vi "GUI PJVS setup.vi"(10 "SS measurement":T1={"Signal frequencies (Hz)"=[1000.0], "Signal amplitudes (V)"=[0.707], "Sampling frequencies (Hz)"=[10000000.0], "Record lengths (multiples of periods)"=[10000.0], "Calculate results"=FALSE, "Algorithm"="TWM-WFFT", "TWM data directories"=[], "TWM data directories relative"=[], "Settle down after AC source change (s)"=1.0, "PJVS frequencies (Hz)"=[1000.0], "PJVS reference voltages array of vector cluster"=[{"PJVS reference voltages vector"=[]}], "Requested PJVS steps"=[20], "Measure CE"=FALSE, "Measure CE before"=FALSE, "Measure CE after"=FALSE, "Single point CE measurement"=FALSE, "original CE template path"=path "", "new CE template path before SS"=path "", "new CE template path before SS relative"=path "", "new CE template path after SS"=path "", "new CE template path after SS relative"=path "", "original CE fit path"=path "", "new CE fit path before SS"=path "", "new CE fit path before SS relative"=path "", "new CE fit path after SS"=path "", "new CE fit path after SS relative"=path "", "Measure digitizer gain"=FALSE, "Measure digitizer gain before"=FALSE, "Measure digitizer gain after"=FALSE, "Digitizer gain"=0.0, "Data folder"=path "", "FR fit path"=path "", "new FR fit path relative"=path "", "Rs"=0, "Re"=0, "SS measurement info files"=[]} {"PJVS reference voltages array of vector cluster"."PJVS reference voltages vector" format="%#_3p"; "PJVS frequencies (Hz)" format="%#_3p"; "Record lengths (multiples of periods)" format="%#_3p"; "Sampling frequencies (Hz)" format="%#_3p"; "Signal amplitudes (V)" format="%#_3p"; "Signal frequencies (Hz)" format="%#_3p"}, 11 "PJVS":T2={"PJVS type"=enum."AC-supraVOLTcontrol", "Status Refnum"=refnum, "AC-supraVOLTcontrol"={"IP address:port (0.0.0.0:0000)"="0.0.0.0:0000", "Timeouts"={"TCP Read & Write (ms)"=7000, "Sensors readout"=5000, "PJVS setup"=10000, "Nullmeter readout"=5000, "Multiplexer setup"=3000, "57XX setup"=15000, "Generator setup"=5000, "Synthesizer setup"=3000, "Sampler readout"=10000}, "Simulation mode"=FALSE, "Debug mode"=FALSE}, "NPL bias source"={"DataSocketCluster"={"Server Machine"="CZC", "Client Machine"="localhost", "Data"="P2", "TimeStamp"=0.0, "Count"=1, "Target Process"="General Server"}}, "Manual PJVS"={"PJVS frequency (Hz)"=0.0, "Reference voltages (V)"=[], "File with PJVS voltages"=path ""}, "VTT PJVS"={"some VTT only property"=""}} {"NPL bias source"."DataSocketCluster"."TimeStamp" format="%.2f"}) -> (2 "SS measurement out":T1={"Signal frequencies (Hz)"=[1000.0], "Signal amplitudes (V)"=[0.707], "Sampling frequencies (Hz)"=[10000000.0], "Record lengths (multiples of periods)"=[10000.0], "Calculate results"=FALSE, "Algorithm"="TWM-WFFT", "TWM data directories"=[], "TWM data directories relative"=[], "Settle down after AC source change (s)"=1.0, "PJVS frequencies (Hz)"=[1000.0], "PJVS reference voltages array of vector cluster"=[{"PJVS reference voltages vector"=[]}], "Requested PJVS steps"=[20], "Measure CE"=FALSE, "Measure CE before"=FALSE, "Measure CE after"=FALSE, "Single point CE measurement"=FALSE, "original CE template path"=path "", "new CE template path before SS"=path "", "new CE template path before SS relative"=path "", "new CE template path after SS"=path "", "new CE template path after SS relative"=path "", "original CE fit path"=path "", "new CE fit path before SS"=path "", "new CE fit path before SS relative"=path "", "new CE fit path after SS"=path "", "new CE fit path after SS relative"=path "", "Measure digitizer gain"=FALSE, "Measure digitizer gain before"=FALSE, "Measure digitizer gain after"=FALSE, "Digitizer gain"=0.0, "Data folder"=path "", "FR fit path"=path "", "new FR fit path relative"=path "", "Rs"=0, "Re"=0, "SS measurement info files"=[]} {"PJVS reference voltages array of vector cluster"."PJVS reference voltages vector" format="%#_3p"; "PJVS frequencies (Hz)" format="%#_3p"; "Record lengths (multiples of periods)" format="%#_3p"; "Sampling frequencies (Hz)" format="%#_3p"; "Signal amplitudes (V)" format="%#_3p"; "Signal frequencies (Hz)" format="%#_3p"}, 3 "PJVS out":T2={"PJVS type"=enum."AC-supraVOLTcontrol", "Status Refnum"=refnum, "AC-supraVOLTcontrol"={"IP address:port (0.0.0.0:0000)"="0.0.0.0:0000", "Timeouts"={"TCP Read & Write (ms)"=7000, "Sensors readout"=5000, "PJVS setup"=10000, "Nullmeter readout"=5000, "Multiplexer setup"=3000, "57XX setup"=15000, "Generator setup"=5000, "Synthesizer setup"=3000, "Sampler readout"=10000}, "Simulation mode"=FALSE, "Debug mode"=FALSE}, "NPL bias source"={"DataSocketCluster"={"Server Machine"="CZC", "Client Machine"="localhost", "Data"="P2", "TimeStamp"=0.0, "Count"=1, "Target Process"="General Server"}}, "Manual PJVS"={"PJVS frequency (Hz)"=0.0, "Reference voltages (V)"=[], "File with PJVS voltages"=path ""}, "VTT PJVS"={"some VTT only property"=""}} {"NPL bias source"."DataSocketCluster"."TimeStamp" format="%.2f"})   [LabVIEW 2020]
doc: "Use this template to build a producer/consumer design pattern with events to produce queue items. Use this design pattern instead of the User Interface Event Handler pattern for user interfaces when you want to execute code asynchronously in response to an event without slowing the user interface responsiveness."
uses:
  General PJVS driver/Type definitions/PJVS.ctl
  General PJVS driver/Type definitions/PJVS Type.ctl
  external libraries/acsvcontrol-driver/Public/Type Definitions/Timeouts.ctl
  external libraries/JV modified NPL Bias source/DataSocketCluster external.ctl
  SS Measurement/Type definitions/SS measurement.ctl
  <vilib>/Utility/error.llb/Error Cluster From Error Code.vi
  <vilib>/Utility/file.llb/Read Delimited Spreadsheet (DBL).vi
  <vilib>/ErrorRing/Error Ring.xnode
  external libraries/varilib/varilib.lvlib
  external libraries/acsvcontrol-driver/ACSVcontrol-driver.lvlib
panel:
  out "gui_elements":refnum<vi>[](array[refnum])
  out "Status":string
  out "error out":errorcluster
  in  "save_and_quit":bool
  in  "PJVS type tab":T6(tab)
  in  "Debug mode":bool
  in  "IP address:port (0.0.0.0:0000)":string
  in  "Timeouts":T4={"TCP Read & Write (ms)"=7000, "Sensors readout"=5000, "PJVS setup"=5000, "Nullmeter readout"=5000, "Multiplexer setup"=3000, "57XX setup"=15000, "Generator setup"=5000, "Synthesizer setup"=3000, "Sampler readout"=10000}
  in  "Simulation mode":bool
  out "DataSocketCluster":T5 {"TimeStamp" format="%.2f"}
  out "manual: no of voltages":i32 caption="Number of reference voltages in the table"
  in  "File with PJVS voltages":path caption="File with reference voltages"
  in  "load voltages":bool
  in  "manual: reference voltages (V)":dbl[](array[numeric]) caption="Reference voltages (V)\n(voltages of PJVS steps)" format="%0.12g"
  in  "Set PJVS frequency (Hz)":dbl caption="PJVS frequency (Hz)\n(frequency of one PJVS period)" format="%#_9g"
  in  "test":bool
  in  "cancel":bool
  # "For testing, either select Manual PJVS, or set \"AC-supraVOLTcontrol\" and\nset \"Simulation mode\". In this way this software can be tested without running a real PJVS."
  # "Manual mode help\nEither enter reference voltages manually into the table, or select a file and load it using the button. The file must be a text file with PJVS values in a first collumn of a tab or comma separated table.\n\nDo not forget to set PJVS frequency."
  # "#VTT add something here"
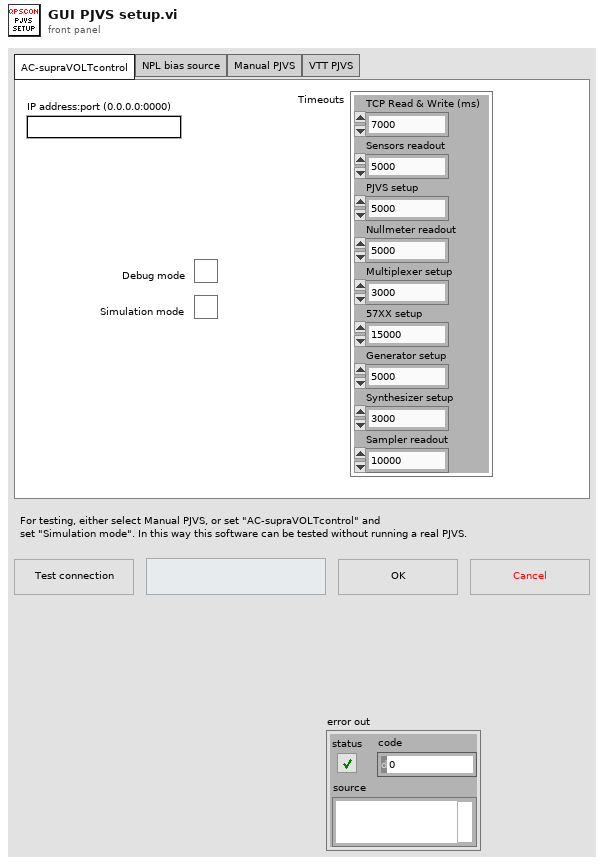
[diagram p1: front panel]
types:
  T1 = typedef "SS measurement.ctl" = cluster{"Signal frequencies (Hz)":dbl[], "Signal amplitudes (V)":dbl[], "Sampling frequencies (Hz)":dbl[], "Record lengths (multiples of periods)":dbl[], "Calculate results":bool, "Algorithm":string, "TWM data directories":path[], "TWM data directories relative":path[], "Settle down after AC source change (s)":dbl, "PJVS frequencies (Hz)":dbl[], "PJVS reference voltages array of vector cluster":cluster{"PJVS reference voltages vector":dbl[]}[], "Requested PJVS steps":u32[], "Measure CE":bool, "Measure CE before":bool, "Measure CE after":bool, "Single point CE measurement":bool, "original CE template path":path, "new CE template path before SS":path, "new CE template path before SS relative":path, "new CE template path after SS":path, "new CE template path after SS relative":path, "original CE fit path":path, "new CE fit path before SS":path, "new CE fit path before SS relative":path, "new CE fit path after SS":path, "new CE fit path after SS relative":path, "Measure digitizer gain":bool, "Measure digitizer gain before":bool, "Measure digitizer gain after":bool, "Digitizer gain":dbl, "Data folder":path, "FR fit path":path, "new FR fit path relative":path, "Rs":i32, "Re":i32, "SS measurement info files":path[]}
  T2 = typedef "PJVS.ctl" = cluster{"PJVS type":T3, "Status Refnum":refnum<vi>, "AC-supraVOLTcontrol":cluster{"IP address:port (0.0.0.0:0000)":string, "Timeouts":T4, "Simulation mode":bool, "Debug mode":bool}, "NPL bias source":cluster{"DataSocketCluster":T5}, "Manual PJVS":cluster{"PJVS frequency (Hz)":dbl, "Reference voltages (V)":dbl[], "File with PJVS voltages":path}, "VTT PJVS":cluster{"some VTT only property":string}}
  T3 = typedef "PJVS Type.ctl" = enum16{"AC-supraVOLTcontrol", "JV modified NPL bias control", "Manual PJVS", "VTT PJVS"}
  T4 = typedef "ACSVcontrol-driver.lvlib/Timeouts.ctl" = cluster{"TCP Read & Write (ms)":i32, "Sensors readout":i32, "PJVS setup":i32, "Nullmeter readout":i32, "Multiplexer setup":i32, "57XX setup":i32, "Generator setup":i32, "Synthesizer setup":i32, "Sampler readout":i32}
  T5 = typedef "DataSocketCluster external.ctl" = cluster{"Server Machine":string, "Client Machine":string, "Data":string, "TimeStamp":dbl, "Count":i32, "Target Process":string}
  T6 = enum32{"AC-supraVOLTcontrol", "NPL bias source", "Manual PJVS", "VTT PJVS"}
  T7 = cluster{"PJVS reference voltages vector":dbl[]}[]
  T8 = cluster{"IP address:port (0.0.0.0:0000)":string, "Timeouts":T4, "Simulation mode":bool, "Debug mode":bool}
  T9 = cluster{"PJVS frequency (Hz)":dbl, "Reference voltages (V)":dbl[], "File with PJVS voltages":path}
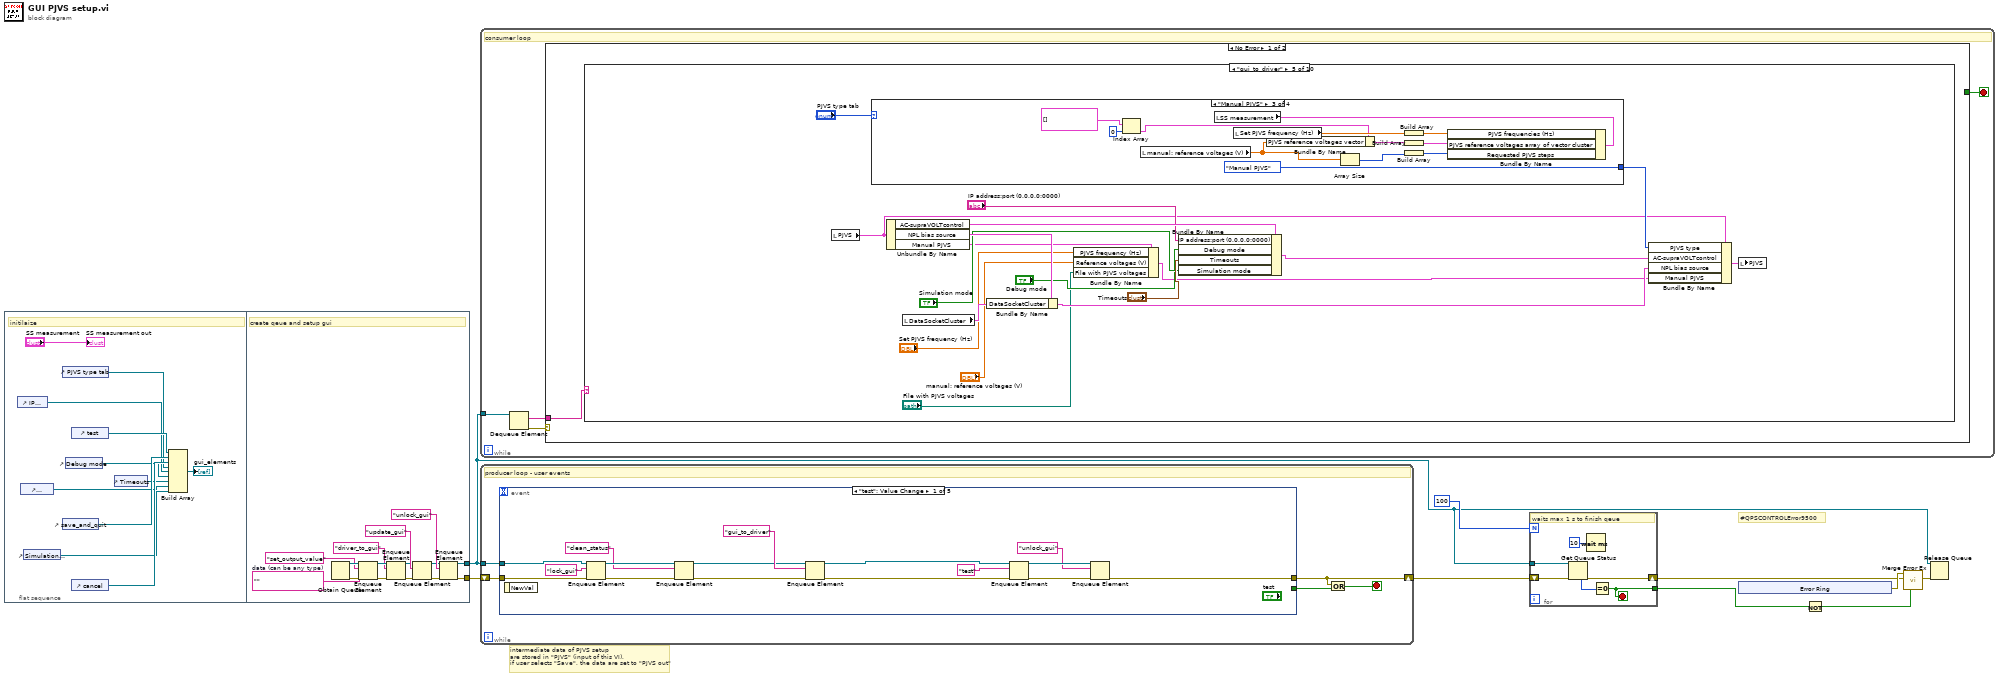
[diagram p0: block diagram]
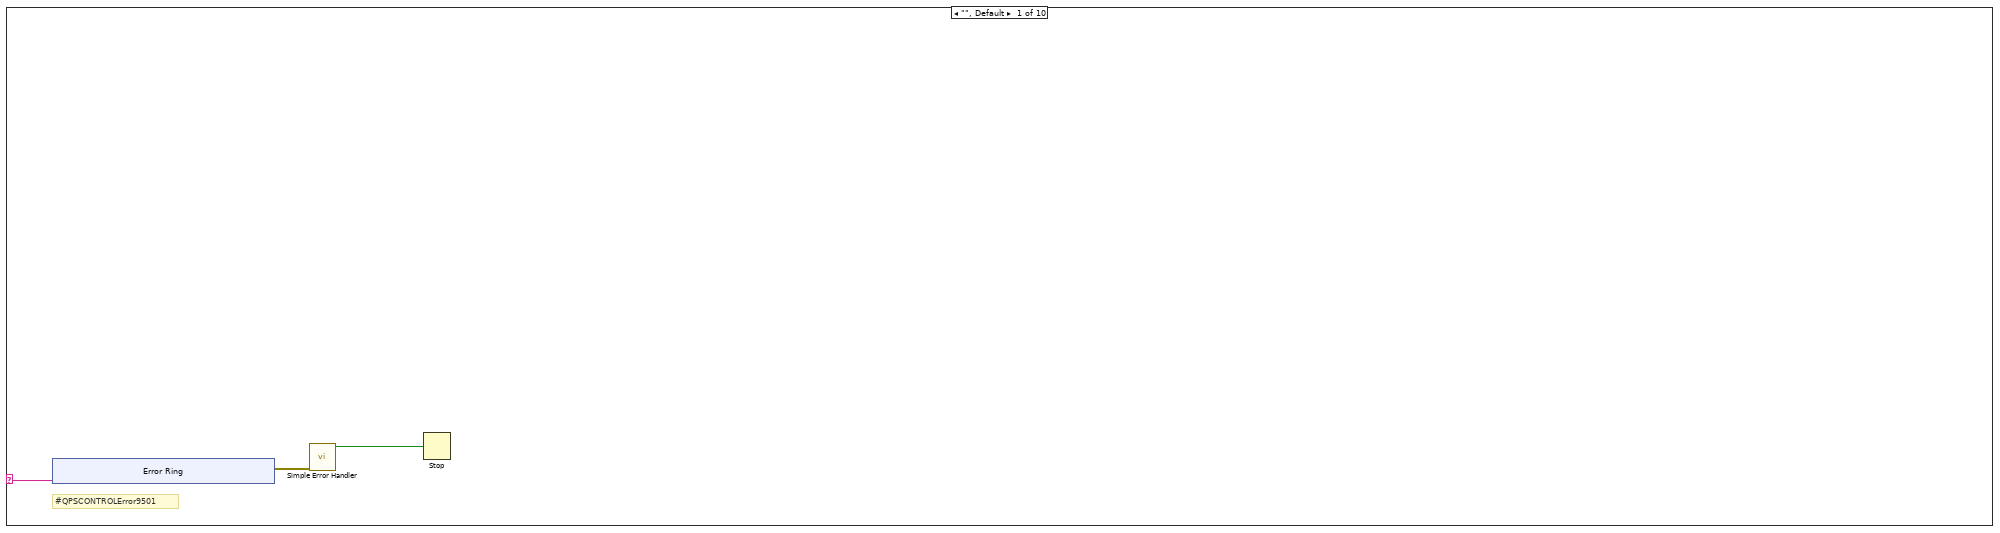
[diagram p2: hidden frame]
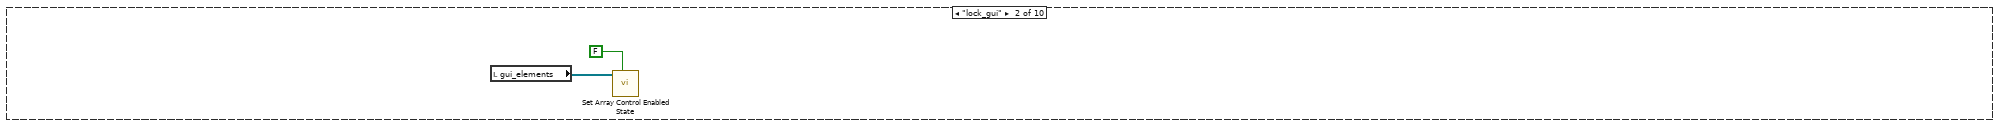
[diagram p3: hidden frame]
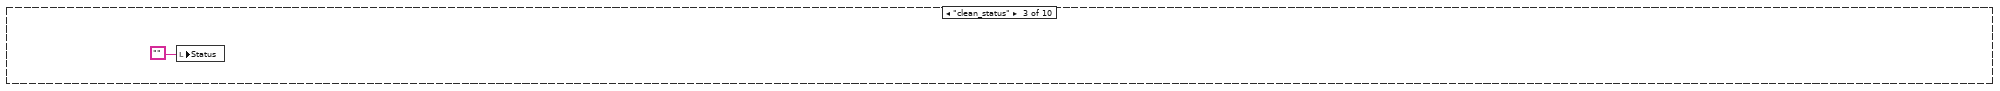
[diagram p4: hidden frame]
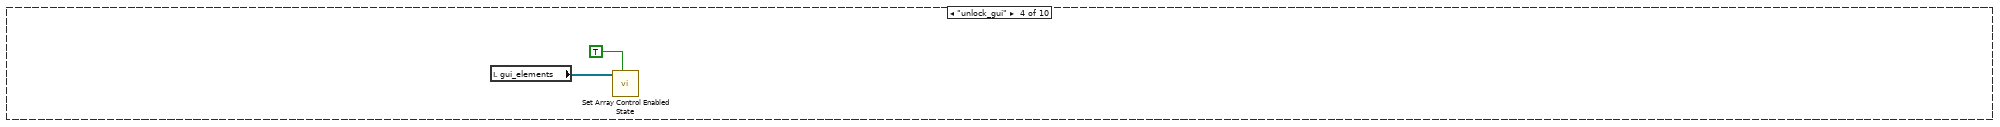
[diagram p5: hidden frame]
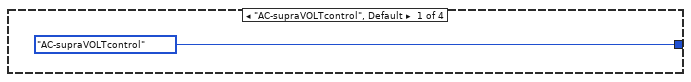
[diagram p6: hidden frame]
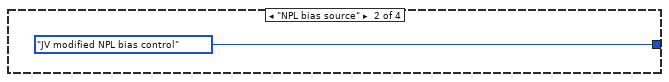
[diagram p7: hidden frame]
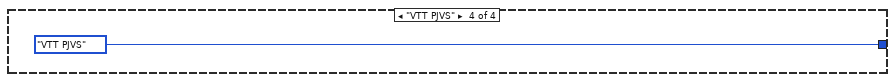
[diagram p8: hidden frame]
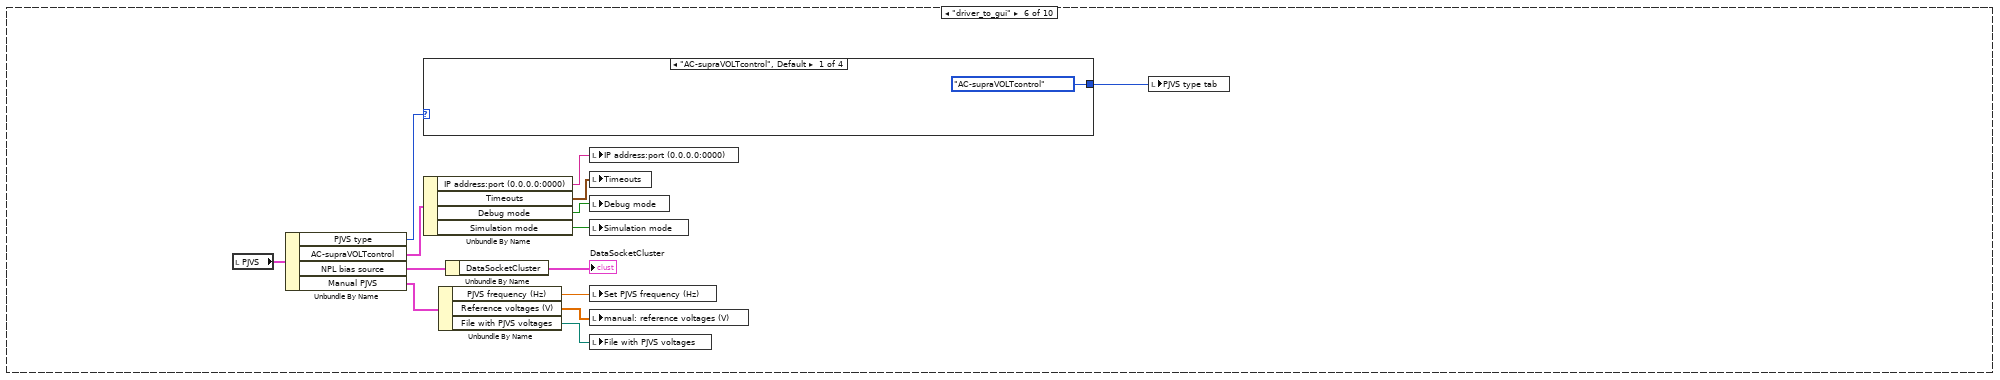
[diagram p9: hidden frame]
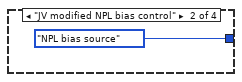
[diagram p10: hidden frame]
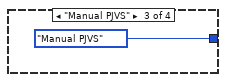
[diagram p11: hidden frame]
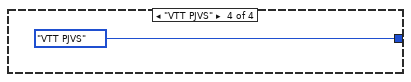
[diagram p12: hidden frame]
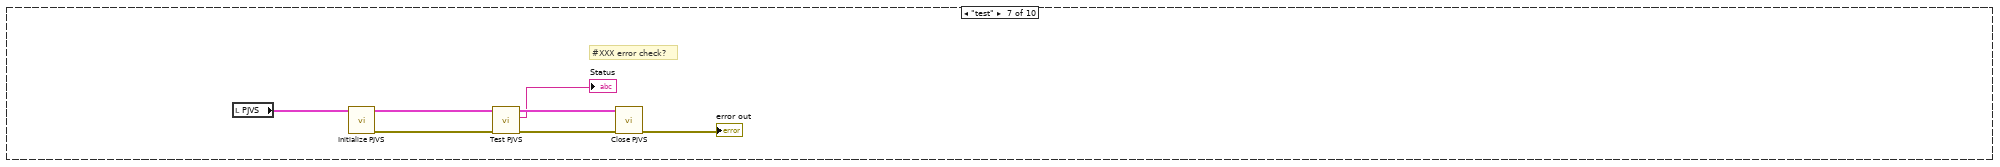
[diagram p13: hidden frame]
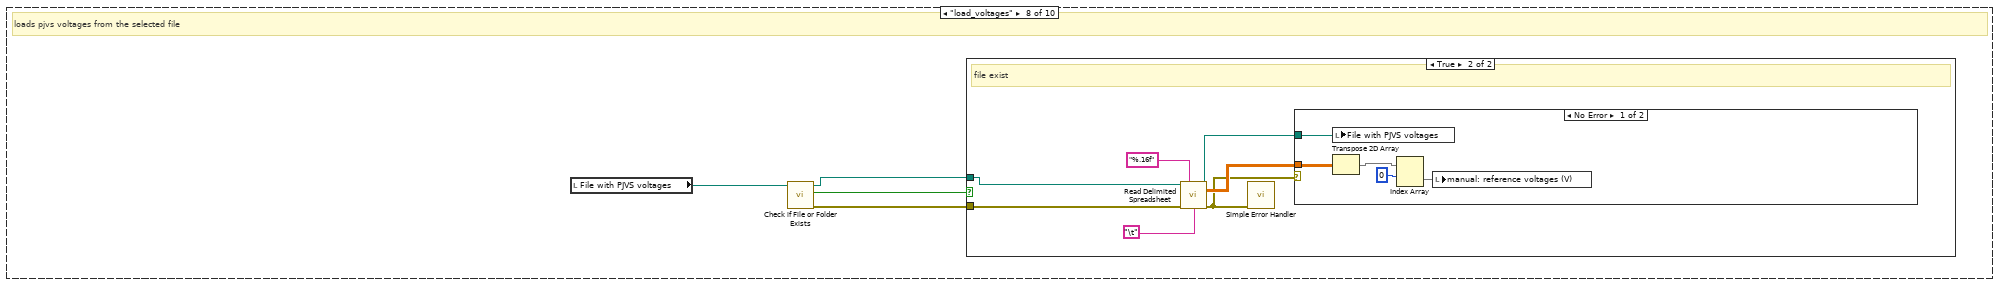
[diagram p14: hidden frame]
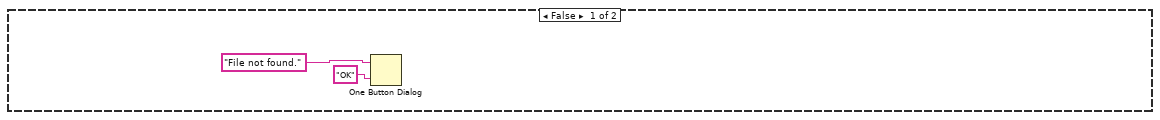
[diagram p15: hidden frame]
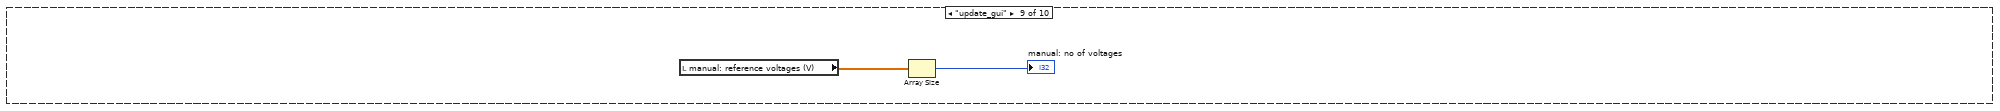
[diagram p17: hidden frame]
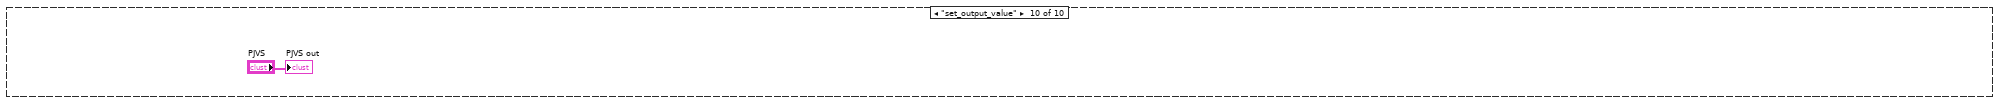
[diagram p18: hidden frame]
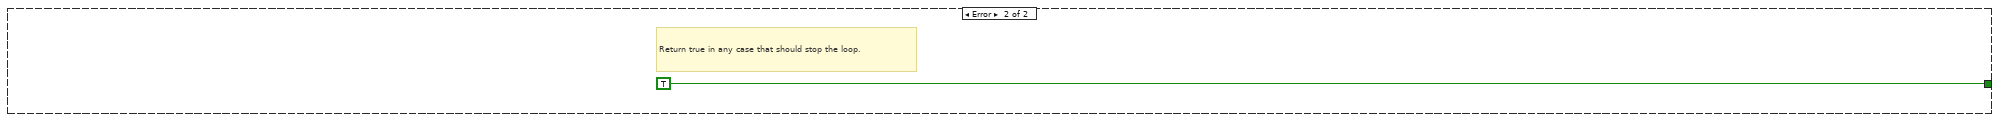
[diagram p19: hidden frame]
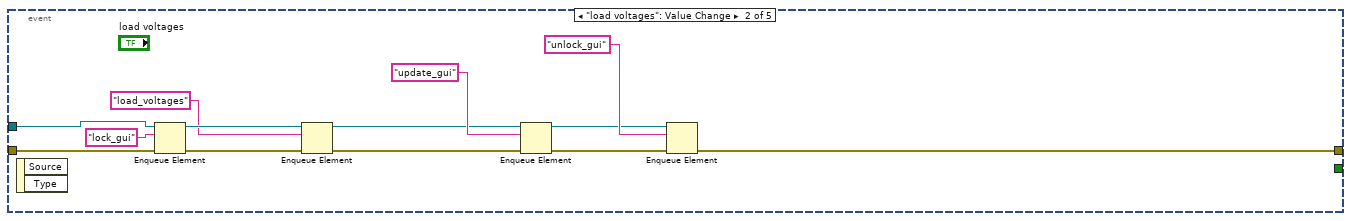
[diagram p20: hidden frame]
diagram:
  # "#QPSCONTROLError9500"
  # "intermediate data of PJVS setup\nare stored in \"PJVS\" (input of this VI),\nif user selects \"Save\", the data are set to \"PJVS out\""
  n1 = flat-sequence {
    tunnel: [w28] -> w2
    tunnel: [w26] -> w1
    frame #0 {
      # "initilaize"
      n2 = control-ref of="IP address:port (0.0.0.0:0000)"() -> (w16:refnum<vi>)
      n3 = control-ref of="DataSocketCluster"() -> (w11:refnum<vi>)
      n4 = control-ref of="Simulation mode"() -> (w13:refnum<vi>)
      n5 = control-ref of="PJVS type tab"() -> (w17:refnum<vi>)
      n6 = control-ref of="save_and_quit"() -> (w19:refnum<vi>)
      n7 = control-ref of="Debug mode"() -> (w12:refnum<vi>)
      n8 = control-ref of="test"() -> (w20:refnum<vi>)
      n9 = control-ref of="cancel"() -> (w18:refnum<vi>)
      n10 = control-ref of="Timeouts"() -> (w15:refnum<vi>)
      n11 = Build Array(w20, w19, w18, w17, w16, w12, w15, w11, w13) -> (→"gui_elements":refnum<vi>[])
      "SS measurement out" <- "SS measurement"
    }
    frame #1 {
      w27 = ""  # data (can be any type)
      # "create qeue and setup gui"
      n12 = Obtain Queue(element data type=w27) -> (queue out=w32:refnum<queue>, error out=w34:errorcluster)  [unwired: 4 in, 1 out]
      n13 = Enqueue Element(queue=w32, element="set_output_value", error in (no error)=w34) -> (queue out=w33:refnum<queue>, error out=w35:errorcluster)  [unwired: 1 in, 1 out]
      n14 = Enqueue Element(queue=w33, element="driver_to_gui", error in (no error)=w35) -> (queue out=w24:refnum<queue>, error out=w21:errorcluster)  [unwired: 1 in, 1 out]
      n15 = Enqueue Element(queue=w24, element="update_gui", error in (no error)=w21) -> (queue out=w23:refnum<queue>, error out=w22:errorcluster)  [unwired: 1 in, 1 out]
      n16 = Enqueue Element(queue=w23, element="unlock_gui", error in (no error)=w22) -> (queue out=w28:refnum<queue>, error out=w26:errorcluster)  [unwired: 1 in, 1 out]
    }
  }
  n17 = while {
    tunnel: w2 -> [w39]
    stop <- w36 stop-if-true
    # "consumer loop"
    n18 = Dequeue Element(queue=w39) -> (element=w37:string, error out=w38:errorcluster)  [unwired: 2 in, 2 out]
    n19 = case shown="No Error" w38 {
      tunnel: w37 -> [w40 _]
      tunnel: [_ TRUE] -> w36
      frame No Error {
        n20 = case shown="\"gui_to_driver\"" w40 {
          selector: w40 -> [w41 _ _ _ _ _ _ _ _ _]
          frame "", Default {
            # "#QPSCONTROLError9501"
            n21 = xnode "Error Ring"("parameter 0"=w41) -> ("error out"=w43:errorcluster)
            n22 = call <vilib>:"Simple Error Handler.vi"("error in (no error)"=w43) -> ("error?"=w42:bool)  [unwired: 4 in, 4 out]
            n23 = Stop(stop? (T)=w42) -> ()
          }
          frame "lock_gui" {
            n24 = local read "gui_elements"() -> (w52:refnum<vi>[])
            n25 = call "Set Array Control Enabled State.vi"("enabled (T)"=FALSE, "reference array in"=w52) -> ()  [unwired: 8 in, 2 out]
          }
          frame "clean_status" {
            n26 = local write "Status"("") -> ()
          }
          frame "unlock_gui" {
            n27 = local read "gui_elements"() -> (w55:refnum<vi>[])
            n28 = call "Set Array Control Enabled State.vi"("enabled (T)"=TRUE, "reference array in"=w55) -> ()  [unwired: 8 in, 2 out]
          }
          frame "gui_to_driver" {
            n29 = local read "PJVS"() -> (w66:T2)
            n30 = case shown="\"Manual PJVS\"" "PJVS type tab" {
              tunnel: [PJVS_Type."AC-supraVOLTcontrol" ("PJVS type") PJVS_Type."JV modified NPL bias control" ("PJVS type") PJVS_Type."Manual PJVS" ("PJVS type") PJVS_Type."VTT PJVS" ("PJVS type")] -> w71
              frame "AC-supraVOLTcontrol", Default {
              }
              frame "NPL bias source" {
              }
              frame "Manual PJVS" {
                n31 = Index Array(array=T7 [] ("PJVS reference voltages array of vector cluster"), index=0) -> (element=w79:cluster{"PJVS reference voltages vector":dbl[]})
                n32 = local read "manual: reference voltages (V)"() -> (w78:dbl[])
                n33 = local read "SS measurement"() -> (w86:T1)
                n34 = local read "Set PJVS frequency (Hz)"() -> (w85:dbl)
                n35 = Bundle By Name(cluster=w79, "PJVS reference voltages vector"=w78) -> (w77:cluster{"PJVS reference voltages vector":dbl[]})
                n36 = Array Size(array=w78) -> (size(s)=w83:i32)
                n37 = Build Array(w85) -> (w84:dbl[])
                n38 = Build Array(w77) -> (w76:T7)
                n39 = Build Array(w83) -> (w82:i32[])
                n40 = Bundle By Name(cluster=w86, "PJVS frequencies (Hz)"=w84, "PJVS reference voltages array of vector cluster"=w76, "Requested PJVS steps"=w82) -> ()  [unwired: 1 out]
              }
              frame "VTT PJVS" {
              }
            }
            n41 = Unbundle By Name(w66) -> ("AC-supraVOLTcontrol"=w70:T8, "NPL bias source"=w65:cluster{"DataSocketCluster":T5}, "Manual PJVS"=w60:T9)
            n42 = local read "DataSocketCluster"() -> (w61:T5)
            n43 = Bundle By Name(cluster=w65, "DataSocketCluster"=w61) -> (w64:cluster{"DataSocketCluster":T5})
            n44 = Bundle By Name(cluster=w60, "PJVS frequency (Hz)"="Set PJVS frequency (Hz)", "Reference voltages (V)"="manual: reference voltages (V)", "File with PJVS voltages"="File with PJVS voltages") -> (w59:T9)
            n45 = Bundle By Name(cluster=w70, "IP address:port (0.0.0.0:0000)"="IP address:port (0.0.0.0:0000)", "Debug mode"="Debug mode", "Timeouts"="Timeouts", "Simulation mode"="Simulation mode") -> (w69:T8)
            n46 = Bundle By Name(cluster=w66, "PJVS type"=w71, "AC-supraVOLTcontrol"=w69, "NPL bias source"=w64, "Manual PJVS"=w59) -> (w73:T2)
            n47 = local write "PJVS"(w73) -> ()
          }
          frame "driver_to_gui" {
            n48 = local read "PJVS"() -> (w93:T2)
            n49 = Unbundle By Name(w93) -> ("PJVS type"=w102:T3, "AC-supraVOLTcontrol"=w101:T8, "NPL bias source"=w98:cluster{"DataSocketCluster":T5}, "Manual PJVS"=w92:T9)
            n50 = case shown="\"AC-supraVOLTcontrol\", Default" w102 {
              tunnel: [T6."AC-supraVOLTcontrol" ("PJVS type tab") T6."NPL bias source" ("PJVS type tab") T6."Manual PJVS" ("PJVS type tab") T6."VTT PJVS" ("PJVS type tab")] -> w94
              frame "AC-supraVOLTcontrol", Default {
              }
              frame "JV modified NPL bias control" {
              }
              frame "Manual PJVS" {
              }
              frame "VTT PJVS" {
              }
            }
            n51 = Unbundle By Name(w101) -> ("IP address:port (0.0.0.0:0000)"=w100:string, "Timeouts"=w99:T4, "Debug mode"=w96:bool, "Simulation mode"=w97:bool)
            n52 = Unbundle By Name(w92) -> ("PJVS frequency (Hz)"=w90:dbl, "Reference voltages (V)"=w91:dbl[], "File with PJVS voltages"=w89:path)
            n53 = Unbundle By Name(w98) -> ("DataSocketCluster"=→"DataSocketCluster":T5)
            n54 = local write "IP address:port (0.0.0.0:0000)"(w100) -> ()
            n55 = local write "Timeouts"(w99) -> ()
            n56 = local write "Debug mode"(w96) -> ()
            n57 = local write "Simulation mode"(w97) -> ()
            n58 = local write "Set PJVS frequency (Hz)"(w90) -> ()
            n59 = local write "manual: reference voltages (V)"(w91) -> ()
            n60 = local write "File with PJVS voltages"(w89) -> ()
            n61 = local write "PJVS type tab"(w94) -> ()
          }
          frame "test" {
            # "#XXX error check?"
            n62 = local read "PJVS"() -> (w109:T2)
            n63 = call "Initialize PJVS.vi"("PJVS setup"=w109) -> ("error out"=w113:errorcluster, "PJVS setup out"=w110:T2)  [unwired: 9 in]
            n64 = call "Test PJVS.vi"("error in (pass through)"=w113, "PJVS setup"=w110) -> ("error out"=w112:errorcluster, "Status"=→"Status":string, "PJVS setup out"=w111:T2)  [unwired: 7 in]
            n65 = call "Close PJVS.vi"("error in (pass through)"=w112, "PJVS setup"=w111) -> ("error out"=→"error out":errorcluster)  [unwired: 8 in, 1 out]
          }
          frame "load_voltages" {
            # "loads pjvs voltages from the selected file"
            n66 = local read "File with PJVS voltages"() -> (w117:path)
            n67 = call <vilib>:"Check if File or Folder Exists.vi"("path"=w117) -> ("error out"=w115:errorcluster, "file or folder exists?"=w114:bool, "dup path"=w116:path)  [unwired: 8 in]
            n68 = case shown="True" w114 {
              tunnel: w116 -> [_ w123]
              tunnel: w115 -> [_ w122]
              frame False {
                n69 = One Button Dialog(message="File not found.", button name ("OK")="OK") -> ()  [unwired: 1 out]
              }
              frame True {
                # "file exist"
                n70 = call-poly <vilib>:"Read Delimited Spreadsheet.vi"("file path (dialog if empty)"=w123, "format (%.3f)"="%.16f", "error in (no error)"=w122, "delimiter (\\t)"="\t") -> ("new file path (Not A Path if cancelled)"=w121:path, "all rows"=w124:dbl[][], "error out"=w120:errorcluster)  [unwired: 6 in, 3 out]
                n71 = call <vilib>:"Simple Error Handler.vi"("error in (no error)"=w120) -> ()  [unwired: 4 in, 5 out]
                n72 = case shown="No Error" w120 {
                  tunnel: w124 -> [w129 _]
                  tunnel: w121 -> [w127 _]
                  frame No Error {
                    n73 = local write "File with PJVS voltages"(w127) -> ()
                    n74 = Transpose 2D Array(2D array=w129) -> (transposed array=w128:dbl[][])
                    n75 = Index Array(array=w128, index (row)=0 ("index")) -> (element=w130:dbl[])  [unwired: 1 in]
                    n76 = local write "manual: reference voltages (V)"(w130) -> ()
                  }
                  frame Error {
                  }
                }
              }
            }
          }
          frame "update_gui" {
            n77 = local read "manual: reference voltages (V)"() -> (w133:dbl[])
            n78 = Array Size(array=w133) -> (size(s)=→"manual: no of voltages":i32)
          }
          frame "set_output_value" {
            "PJVS out" <- "PJVS"
          }
        }
      }
      frame Error {
        # "Return true in any case that should stop the loop."
      }
    }
  }
  n79 = while {
    shift-right: [w136] -> w5
    shift-left: w1 -> [w139]
    tunnel: w2 -> [w140]
    stop <- w137 stop-if-true
    # "producer loop - user events"
    n80 = event shown="[0] \"test\": Value Change" {
      selector: _ -> [_ _ _ _ _]
      dyn-events: _ -> [_ _ _ _ _]
      timeout: _ -> [_ _ _ _ _]
      tunnel: w140 -> [w147 w163 w171 w178 _]
      tunnel: w139 -> [w148 w164 w172 w175 w183]
      tunnel: [w151 w162 w170 w174 w183] -> w136
      tunnel: [_ _ _ TRUE ("cancel") TRUE ("cancel")] -> w138
      event "test": Value Change {
        n81 = event-data() -> ()  [unwired: 1 in, 1 out]
        n82 = Enqueue Element(queue=w147, element="lock_gui", error in (no error)=w148) -> (queue out=w144:refnum<queue>, error out=w145:errorcluster)  [unwired: 1 in, 1 out]
        n83 = Enqueue Element(queue=w144, element="clean_status", error in (no error)=w145) -> (queue out=w142:refnum<queue>, error out=w143:errorcluster)  [unwired: 1 in, 1 out]
        n84 = Enqueue Element(queue=w142, element="gui_to_driver", error in (no error)=w143) -> (queue out=w154:refnum<queue>, error out=w155:errorcluster)  [unwired: 1 in, 1 out]
        n85 = Enqueue Element(queue=w154, element="test", error in (no error)=w155) -> (queue out=w150:refnum<queue>, error out=w152:errorcluster)  [unwired: 1 in, 1 out]
        n86 = Enqueue Element(queue=w150, element="unlock_gui", error in (no error)=w152) -> (error out=w151:errorcluster)  [unwired: 1 in, 2 out]
      }
      event "load voltages": Value Change {
        n87 = event-data() -> ()  [unwired: 1 in, 2 out]
        n88 = Enqueue Element(queue=w163, element="lock_gui", error in (no error)=w164) -> (queue out=w168:refnum<queue>, error out=w169:errorcluster)  [unwired: 1 in, 1 out]
        n89 = Enqueue Element(queue=w168, element="load_voltages", error in (no error)=w169) -> (queue out=w159:refnum<queue>, error out=w160:errorcluster)  [unwired: 1 in, 1 out]
        n90 = Enqueue Element(queue=w159, element="update_gui", error in (no error)=w160) -> (queue out=w158:refnum<queue>, error out=w157:errorcluster)  [unwired: 1 in, 1 out]
        n91 = Enqueue Element(queue=w158, element="unlock_gui", error in (no error)=w157) -> (error out=w162:errorcluster)  [unwired: 1 in, 2 out]
      }
      event "manual: reference voltages (V)": Value Change {
        n92 = event-data() -> ()  [unwired: 1 in, 2 out]
        n93 = Enqueue Element(queue=w171, element="update_gui", error in (no error)=w172) -> (error out=w170:errorcluster)  [unwired: 1 in, 2 out]
      }
      event "save_and_quit": Value Change {
        n94 = event-data() -> ()  [unwired: 1 in, 1 out]
        n95 = Enqueue Element(queue=w178, element="gui_to_driver", error in (no error)=w175) -> (queue out=w177:refnum<queue>, error out=w176:errorcluster)  [unwired: 1 in, 1 out]
        n96 = Enqueue Element(queue=w177, element="set_output_value", error in (no error)=w176) -> (error out=w174:errorcluster)  [unwired: 1 in, 2 out]
      }
      event "cancel": Value Change; Panel Close {
        n97 = event-data() -> ()  [unwired: 1 in, 2 out]
      }
    }
    n98 = Or(x=w136, y=w138) -> (x .or. y?=w137:bool)
  }
  n99 = for {
    N: 100 -> [_]
    tunnel: w2 -> [w189]
    shift-right: [w187] -> w6
    shift-left: w5 -> [w188]
    tunnel: [w184] -> w3
    stop <- w184 stop-if-true
    # "waits max 1 s to finish qeue"
    n100 = Get Queue Status(queue=w189, error in (no error)=w188) -> (error out=w187:errorcluster, # elements in queue=w185:i32)  [unwired: 1 in, 6 out]
    n101 = Wait (ms)(milliseconds to wait=u32 10) -> ()  [unwired: 1 out]
    n102 = Equal To 0?(x=w185) -> (x = 0?=w184:bool)
  }
  n103 = xnode "Error Ring"() -> ("error out"=w7:errorcluster)
  n104 = Not(x=w3) -> (.not. x?=w8:bool)
  n105 = call "Merge Error Ex.vi"("Is error? (False)"=w8, "main error in (no error)"=w6, "second error in"=w7) -> ("error out"=w4:errorcluster)  [unwired: 8 in]
  n106 = Release Queue(queue=w2, error in (no error)=w4) -> ()  [unwired: 1 in, 3 out]
